vi "Point_Set_Timestamp.vi"(6 "Timestamp":timestamp, 8 "Error In":errorcluster, 10 "Tag":string, 11 "Map":T1) -> (0 "Error Out":errorcluster, 3 "Map Out":T1)   [LabVIEW 2017, in "PointValueMap.lvlib"]
doc: "Sets a date and time attribute for a map point. The Point Read VI returns this timestamp if you set one."
uses:
  <vilib>/addons/PointValueMap/PointValueMap.lvlib
  <vilib>/addons/PointValueMap/controls/PointMap.ctl
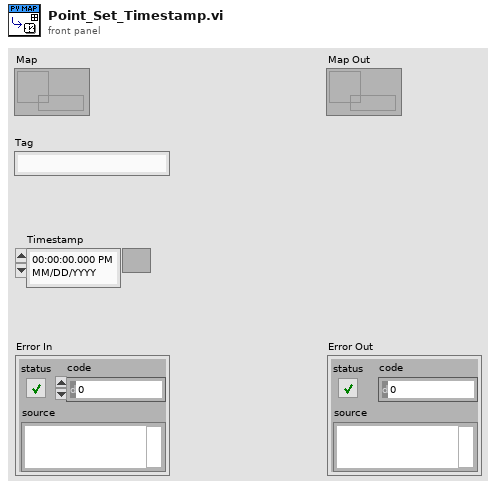
[diagram p1: front panel]
types:
  T1 = typedef "PointValueMap.lvlib/PointMap.ctl" = refnum<data-value>
  T2 = typedef "PointValueMap.lvlib/Point.ctl" = cluster{"Datatype":T3, "Timestamp":timestamp, "Value":variant, "Valid":bool}
  T3 = typedef "PointValueMap.lvlib/DataTypes.ctl" = enum16{"single", "double", "i32", "string", "variant"}
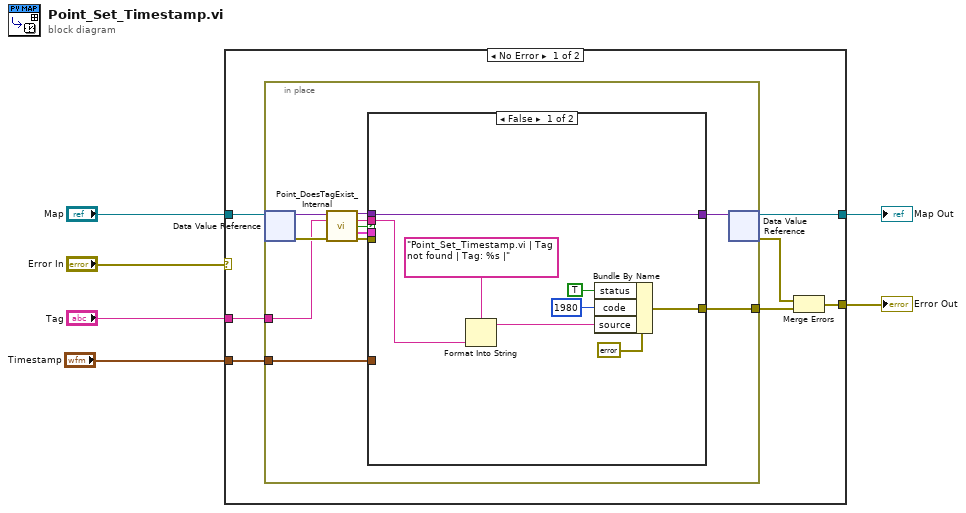
[diagram p0: block diagram]
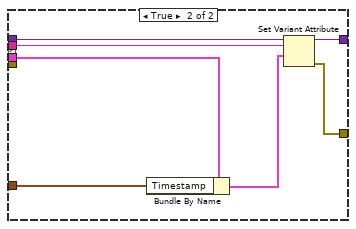
[diagram p2: hidden frame]
diagram:
  n1 = case shown="No Error" "Error In" {
    selector: "Error In" -> [_ w41]
    tunnel: "Map" -> [w13 w40]
    tunnel: "Tag" -> [w12 _]
    tunnel: [w9 w41] -> w5
    tunnel: [w8 w40] -> w2
    tunnel: "Timestamp" -> [w7 _]
    frame No Error {
      n2 = in-place {
        in-place-border: w12 -> [w17]
        in-place-border: [w23] -> w10
        in-place-border: w7 -> [w14]
        n3 = in-place-dvr #1(w13) -> (w22:variant, w20:errorcluster)
        n4 = call <vilib>:"Point_DoesTagExist_Internal.vi"("Map"=w22, "Tag"=w17, "Error In"=w20) -> ("Map Out"=w21:variant, "Tag Out"=w15:string, "Tag Exists"=w18:bool, "Point"=w16:T2, "Error Out"=w19:errorcluster)  [unwired: 7 in, 1 out]
        n5 = case shown="False" w18 {
          tunnel: [w26 w39] -> w24
          tunnel: [w27 w38] -> w23
          tunnel: w21 -> [w26 w37]
          tunnel: w19 -> [_ _]
          tunnel: w16 -> [_ w33]
          tunnel: w15 -> [w25 w36]
          tunnel: w14 -> [_ w34]
          frame False {
            n6 = Format Into String(format string="Point_Set_Timestamp.vi | Tag not found | Tag: %s |" ("source"), w25) -> (resulting string=w29:string)  [unwired: 2 in, 1 out]
            n7 = Bundle By Name(cluster=errorcluster {"status"=FALSE, "code"=0, "source"=""} ("Error Out"), "status"=TRUE, "code"=1980, "source"=w29) -> (w27:errorcluster)
          }
          frame True {
            n8 = Bundle By Name(cluster=w33, "Timestamp"=w34) -> (w35:T2)
            n9 = Set Variant Attribute(Variant=w37, name=w36, value=w35) -> (Variant out=w39:variant, error out=w38:errorcluster)  [unwired: 1 in, 1 out]
          }
        }
        n10 = in-place-dvr #1(w24) -> (w8:T1, w11:errorcluster)
      }
      n11 = Merge Errors(w11, w10) -> (w9:errorcluster)
    }
    frame Error {
    }
  }
  "Error Out" <- w5
  "Map Out" <- w2
